vi "RIMAS Check Detector Controller Status.vi"(8 "error in (no error)":errorcluster, 11 "Detector Ref  in":refnum<k5>) -> (0 "error out":errorcluster, 1 "Status Controllers":string, 2 "Status Headers":string, 3 "Detector Ref out":refnum<k5>)   [LabVIEW 2022 SP3]
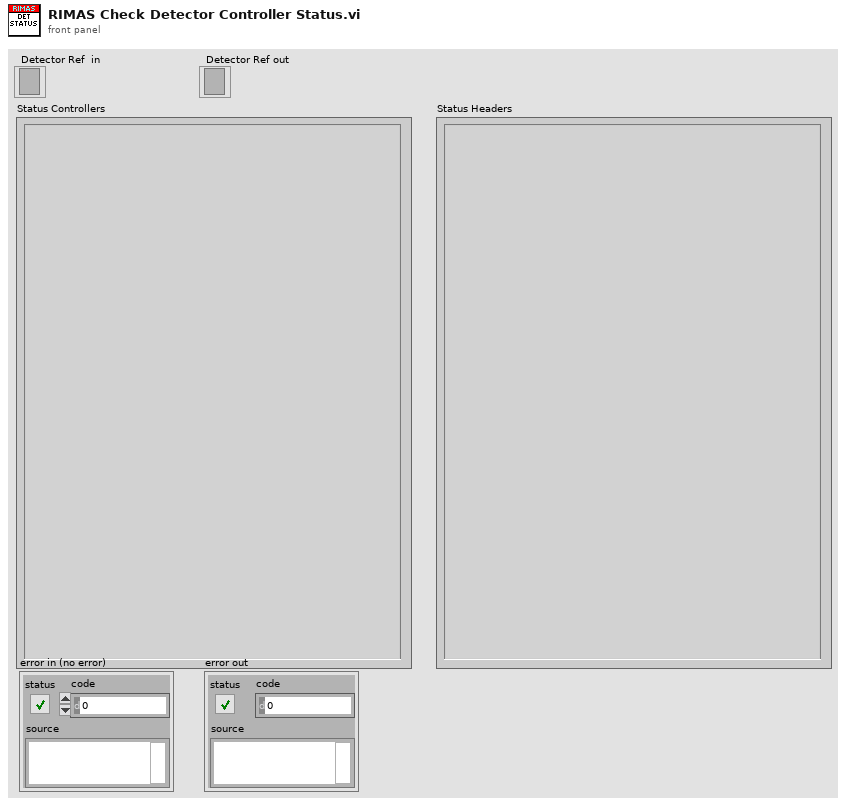
[diagram p1: front panel]
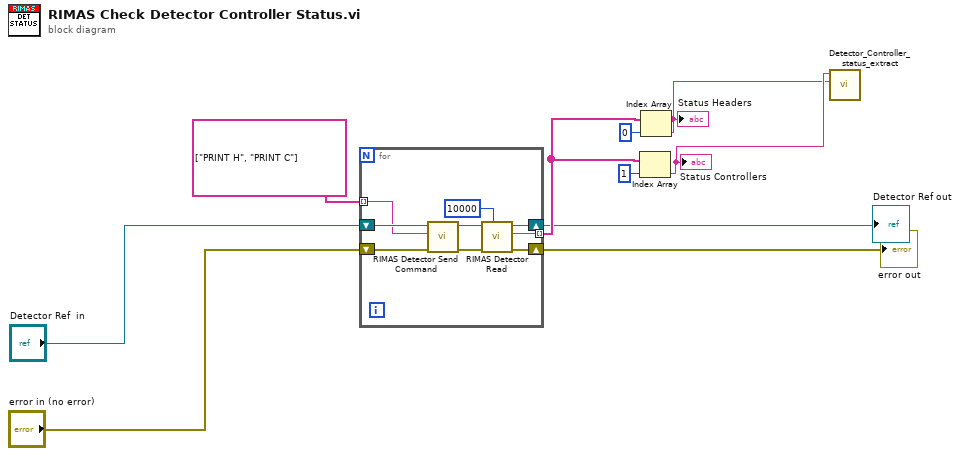
[diagram p0: block diagram]
diagram:
  n1 = for {
    tunnel: [w12] -> w10 mode=indexing
    shift-right: [w16] -> w4
    shift-left: "error in (no error)" -> [w17]
    shift-right: [w13] -> w6
    shift-left: "Detector Ref  in" -> [w14]
    tunnel: string[] ["PRINT H", "PRINT C"] ("Init Commands") -> [w11] mode=indexing
    n2 = call "RIMAS Detector Send Command.vi"("Error In"=w17, "Command"=w11, "Detector Ref"=w14) -> ("Error Out"=w18:errorcluster, "Detector Ref dup"=w19:refnum<k5>)  [unwired: 6 in, 1 out]
    n3 = call "RIMAS Detector Read.vi"("timeout (ms)"=10000, "Error In"=w18, "Detector Ref"=w19) -> ("Error Out"=w16:errorcluster, "data out"=w12:string, "Detector Ref dup"=w13:refnum<k5>)  [unwired: 5 in, 1 out]
  }
  "Detector Ref out" <- w6
  "error out" <- w4
  n4 = Index Array(array=w10, index=1) -> (element=w2:string)
  "Status Controllers" <- w2
  n5 = Index Array(array=w10, index=0) -> (element=w1:string)
  "Status Headers" <- w1
  n6 = call "Detector_Controller_status_extract.vi"("Status Headers"=w1, "Status Controllers"=w2) -> ()  [unwired: 8 in, 2 out]
